vi "Initialize.vi"(8 "error in":errorcluster, 10 "VI Refnum":refnum<vi>, 11 "ManageControls in":refnum<class "Controls_Mgr.lvclass">) -> (0 "error out":errorcluster, 3 "ManageControls out":refnum<class "Controls_Mgr.lvclass">)   [LabVIEW 2015, in "Generic Module Library.lvlib" / "Template G_Module.lvlib" / "Controls_Mgr.lvclass"]
uses:
  Controls_Mgr.lvclass
  <vilib>/Utility/traverseref.llb/VI Scripting - Traverse.lvlib
  <vilib>/Utility/traverseref.llb/TRef TravTarget.ctl
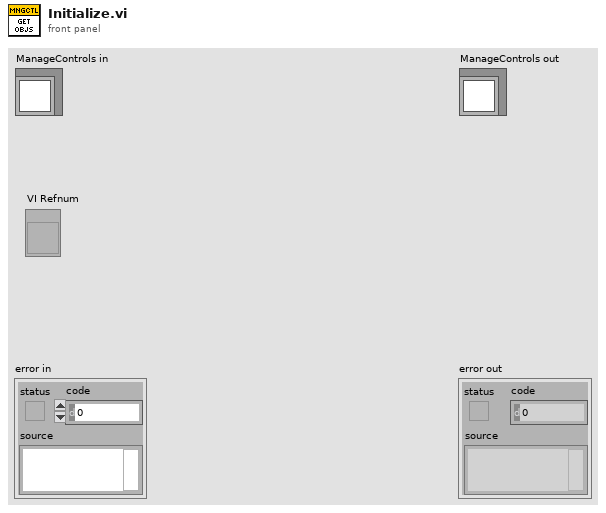
[diagram p1: front panel]
types:
  T1 = typedef "TRef TravTarget.ctl" = enum16{"FP", "BD", "Other"}
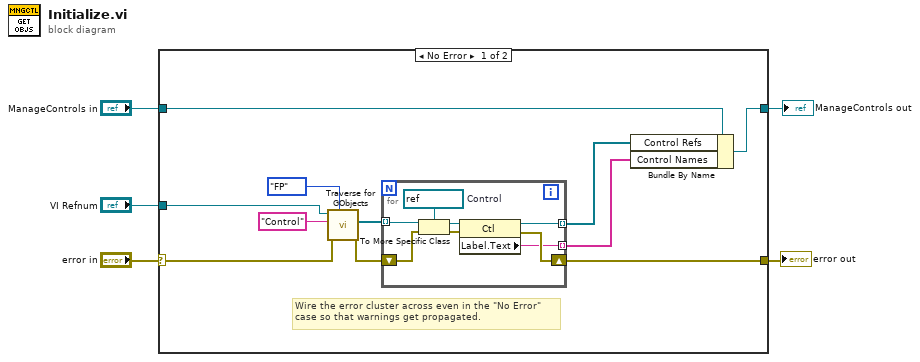
[diagram p0: block diagram]
diagram:
  n1 = case shown="No Error" "error in" {
    selector: "error in" -> [w7 w26]
    tunnel: [w9 w26] -> w4
    tunnel: [w12 w25] -> w2
    tunnel: "ManageControls in" -> [w13 w25]
    tunnel: "VI Refnum" -> [w6 _]
    frame No Error {
      # "Wire the error cluster across even in the \"No Error\"\ncase so that warnings get propagated."
      n2 = call <vilib>:"Traverse for GObjects.vi"("Traverse Target"=TRef_TravTarget."FP", "error in (no error)"=w7, "Class Name"="Control", "VI Refnum"=w6) -> ("error out"=w8:errorcluster, "References"=w14:refnum<vi>[])  [unwired: 4 in, 2 out]
      n3 = for {
        tunnel: w14 -> [w24] mode=indexing
        shift-right: [w20] -> w9
        shift-left: w8 -> [w23]
        tunnel: [w19] -> w11 mode=indexing
        tunnel: [w18] -> w10 mode=indexing
        w17 = refnum<vi> refnum  # Control
        n4 = To More Specific Class(target class=w17, reference=w24, error in=w23) -> (specific class reference=w22:refnum<vi>, error out=w21:errorcluster)
        n5 = property class="Ctl"(reference=w22, error in=w21) -> (reference out=w19:refnum<vi>, error out=w20:errorcluster, "Label.Text"=w18:string)
      }
      n6 = Bundle By Name(cluster=w13, "Control Refs"=w11, "Control Names"=w10) -> (w12:refnum<class "Controls_Mgr.lvclass">)
    }
    frame Error {
    }
  }
  "error out" <- w4
  "ManageControls out" <- w2
